vi "RFSG List Mode Test Signal Generation for 5668.vi"(0 "Resource Name":refnum<k15>="RFSG" caption="resource name", 5 "Start Frequency":dbl=3850000000.0 format="%#_6p", 7 "End Frequency":dbl=4800000000.0 format="%#_6p", 11 "error in (no error)":errorcluster) -> (4 "# Tones":i32, 15 "error out":errorcluster)   [LabVIEW 2017]
doc: "Demonstrates how to create a Configuration List for sweeping frequency and/or power."
uses:
  <instrlib>/niRFSG/niRFSG.llb/niRFSG Ref Clock Sources.ctl
  <instrlib>/niRFSG/niRFSG.llb/niRFSG Configuration List Properties.ctl
  <vilib>/Analysis/1siggen.llb/Ramp Pattern by Delta.vi
  <vilib>/Analysis/NI_AALBase.lvlib
panel:
  in  "delta":dbl=50000000.0 format="%#_6p"
  out "Ramp Pattern":dbl[](array[numeric]) format="%#_6p"
  in  "Power Level (dBm)":dbl format="%_3f"
  in  "Timer:Interval":dbl
  in  "List Trigger Source":string(combo)="PXI_Trig1"
  out "Current Frequency (Hz)":dbl format="%#.3p"
  in  "Frequency Settling (ppm)":dbl=1.0 format="%#.6f"
  in  "Stop":bool
  in  "Reference Clock Source":T1="OnboardClock"
  # "Overview: Demonstrates how to create a Configuration List for sweeping frequency and/or power.\nRequirements: NI-RFSG\nInstructions:\n1. Change the Resource Name to your device.\n2. Run the VI.\n3. Click Stop to stop the VI."
  # "You can set the Start Frequency and End Frequency parameters to the same value to keep the Frequency or Power Level constant."
  # "In order to configure new settings, you must stop the example using \nthe Stop button and then run the VI with the new settings."
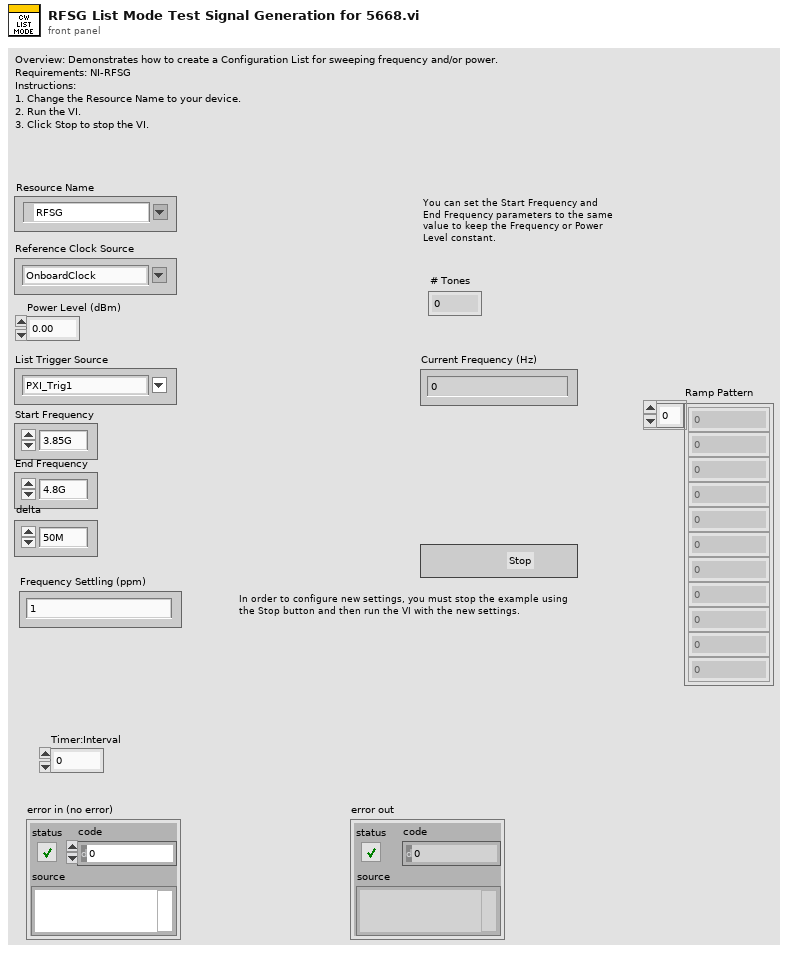
[diagram p1: front panel]
types:
  T1 = typedef "niRFSG Ref Clock Sources.ctl" = string
  T2 = typedef "niRFSG Configuration List Properties.ctl" = u32
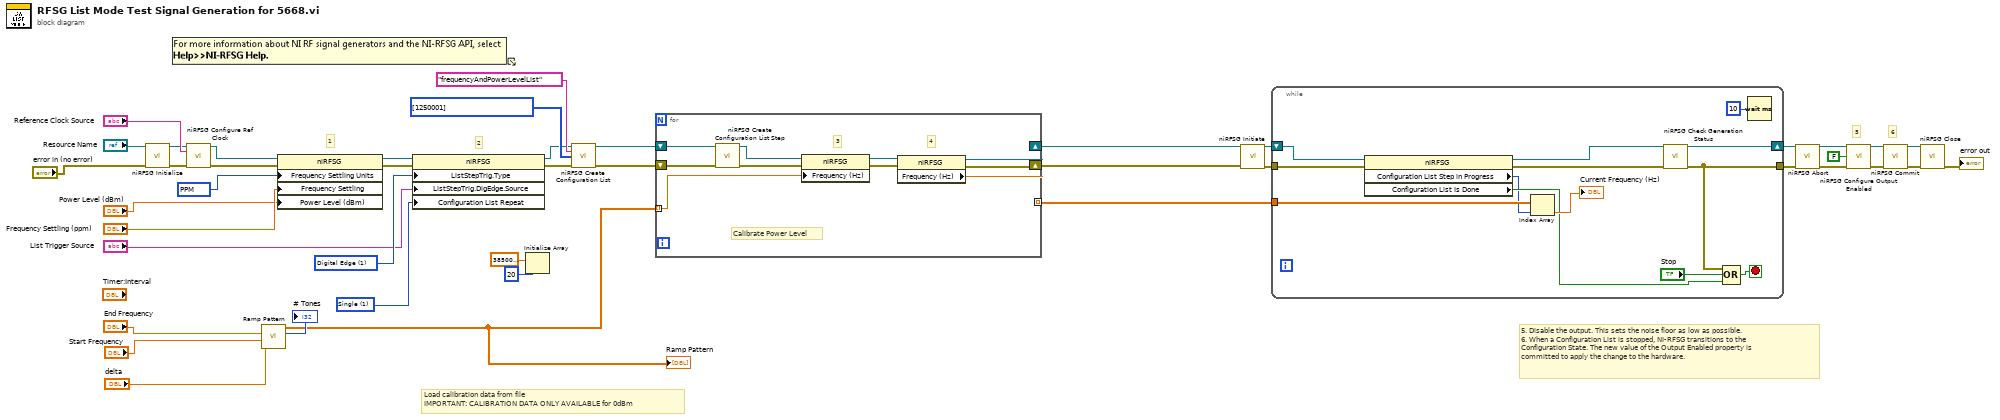
[diagram p0: block diagram]
diagram:
  w8 = 1 items=["Continuous", "Single"] ("Configuration List:Configuration List Repeat")
  w31 = T2[] [1250001] items=["ALC Control"=1150195, "Amp Path"=1150185, "Amplitude Settling (dB)"=1150137, "Attenuator Setting (dB)"=1150173, "Automatic Power Search"=1150196, "Frequency (Hz)"=1250001, "Frequency Settling"=1150083, "IQ Out Port Carrier Frequency"=1150145, "IQ Out Port Common Mode Offset"=1150148, "IQ Out Port Level"=1150147, "IQ Out Port Offset"=1150149, "Output Enabled"=1250004, "Phase Offset (Degrees)"=1150024, "Power Level (dBm)"=1250002, "Pulse Modulation Enabled"=1250051, "Timer Event Interval (s)"=1150100, "Upconverter Center Frequency (Hz)"=1154098] ("configuration list properties")
  w38 = 1 items=["None", "Digital Edge", "Software"] ("Triggers:Configuration List Step:Type")
  w43 = 12002 items=["Seconds After Lock"=12000, "Seconds After I/O"=12001, "PPM"=12002] ("RF:Frequency Settling Units")
  # "Load calibration data from file\nIMPORTANT: CALIBRATION DATA ONLY AVAILABLE for 0dBm"
  # "6"
  # "2"
  # "5. Disable the output. This sets the noise floor as low as possible.\n6. When a Configuration List is stopped, NI-RFSG transitions to the Configuration State. The new value of the Output Enabled property is committed to apply the change to the hardware."
  # "5"
  # "1"
  n1 = call <instrlib>:"niRFSG Initialize.vi"("resource name"="Resource Name", "error in"="error in (no error)") -> ("instrument handle"=w21:refnum<k15>, "error out"=w20:errorcluster)  [unwired: 2 in, 10 out]
  n2 = call <instrlib>:"niRFSG Configure Ref Clock.vi"("instrument handle"=w21, "ref clock source"="Reference Clock Source", "error in"=w20) -> ("instrument handle out"=w10:refnum<k15>, "error out"=w25:errorcluster)  [unwired: 1 in, 10 out]
  n3 = call-poly <vilib>:"Ramp Pattern.vi"("start"="Start Frequency", "end"="End Frequency", "delta"="delta") -> ("samples"=→"# Tones":i32, "Ramp Pattern"=w1:dbl[])  [unwired: 6 in, 1 out]
  "Ramp Pattern" <- w1
  n4 = property class="niRFSG"(reference=w10, error in=w25, "Frequency Settling Units"=w43, "Frequency Settling"="Frequency Settling (ppm)", "Power Level (dBm)"="Power Level (dBm)") -> (reference out=w35:refnum<k15>, error out=w36:errorcluster)
  n5 = property class="niRFSG"(reference=w35, error in=w36, "ListStepTrig.Type"=w38, "ListStepTrig.DigEdge.Source"="List Trigger Source", "Configuration List Repeat"=w8) -> (reference out=w24:refnum<k15>, error out=w32:errorcluster)
  n6 = Initialize Array(3850000000.0 ("element"), 20 ("dimension size")) -> ()  [unwired: 1 out]
  n7 = call <instrlib>:"niRFSG Create Configuration List.vi"("instrument handle"=w24, "list name"="frequencyAndPowerLevelList", "configuration list properties"=w31, "error in"=w32) -> ("instrument handle out"=w18:refnum<k15>, "error out"=w37:errorcluster)  [unwired: 1 in, 9 out]
  n8 = for {
    shift-right: [w48] -> w14
    shift-left: w18 -> [w46]
    shift-right: [w49] -> w13
    shift-left: w37 -> [w45]
    tunnel: [w50] -> w19 mode=indexing
    tunnel: w1 -> [w44] mode=indexing
    # "Calibrate Power Level"
    # "4"
    # "3"
    n9 = call <instrlib>:"niRFSG Create Configuration List Step.vi"("instrument handle"=w46, "error in"=w45) -> ("instrument handle out"=w53:refnum<k15>, "error out"=w47:errorcluster)  [unwired: 1 in, 11 out]
    n10 = property class="niRFSG"(reference=w53, error in=w47, "Frequency (Hz)"=w44) -> (reference out=w52:refnum<k15>, error out=w51:errorcluster)
    n11 = property class="niRFSG"(reference=w52, error in=w51) -> (reference out=w48:refnum<k15>, error out=w49:errorcluster, "Frequency (Hz)"=w50:dbl)
  }
  n12 = call <instrlib>:"niRFSG Initiate.vi"("instrument handle"=w14, "error in"=w13) -> ("instrument handle out"=w41:refnum<k15>, "error out"=w16:errorcluster)  [unwired: 12 out]
  n13 = while {
    shift-right: [w62] -> w39
    shift-left: w41 -> [w61]
    tunnel: w19 -> [w64]
    tunnel: [w60] -> w17
    tunnel: w16 -> [w59]
    stop <- w66 stop-if-true
    n14 = property class="niRFSG"(reference=w61, error in=w59) -> (reference out=w57:refnum<k15>, error out=w58:errorcluster, "Configuration List Step in Progress"=w54:i64, "Configuration List Is Done"=w55:bool)
    n15 = Index Array(array=w64, index=w54) -> (element=→"Current Frequency (Hz)":dbl)
    n16 = call <instrlib>:"niRFSG Check Generation Status.vi"("instrument handle"=w57, "error in"=w58) -> ("instrument handle out"=w62:refnum<k15>, "error out"=w60:errorcluster)  [unwired: 12 out]
    n17 = Compound Arithmetic op=OR(w60, "Stop", w55) -> (w66:bool)
    n18 = Wait (ms)(milliseconds to wait=u32 10) -> ()  [unwired: 1 out]
  }
  n19 = call <instrlib>:"niRFSG Abort.vi"("instrument handle"=w39, "error in"=w17) -> ("instrument handle out"=w23:refnum<k15>, "error out"=w22:errorcluster)  [unwired: 12 out]
  n20 = call <instrlib>:"niRFSG Configure Output Enabled.vi"("instrument handle"=w23, "output enabled"=FALSE ("output enable"), "error in"=w22) -> ("instrument handle out"=w29:refnum<k15>, "error out"=w28:errorcluster)  [unwired: 11 out]
  n21 = call <instrlib>:"niRFSG Commit.vi"("instrument handle"=w29, "error in"=w28) -> ("instrument handle out"=w26:refnum<k15>, "error out"=w27:errorcluster)  [unwired: 12 out]
  n22 = call <instrlib>:"niRFSG Close.vi"("instrument handle"=w26, "error in"=w27) -> ("error out"=→"error out":errorcluster)  [unwired: 13 out]
